vi "Open.vi"(9 "force":dbl, 10 "Lever":refnum<class "Lever.lvclass">, 11 "Box in":refnum<class "Box.lvclass">) -> (3 "Box out":refnum<class "Box.lvclass">)   [LabVIEW 2023, in "Box.lvclass"]
uses:
  Box.lvclass
  c:/dev/_r/4/eng/lv-core/lvpostprocessingd/lv_mc_x86_64/dist_i386/examples/Object-Oriented Programming/Basic Interfaces/Pryable/Pryable.lvclass
  Lever/Lever.lvclass
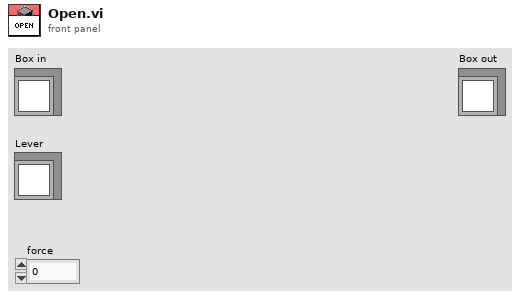
[diagram p1: front panel]
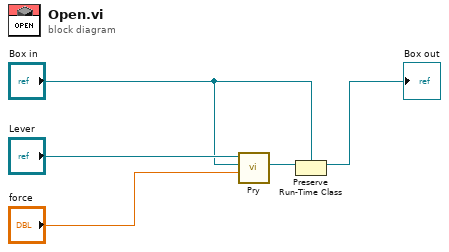
[diagram p0: block diagram]
diagram:
  n1 = call "Pry.vi"("force"="force", "Pryable in"="Box in", "Lever in"="Lever") -> ("Pryable out"=w4:refnum<class "Box.lvclass">)  [unwired: 8 in]
  n2 = Preserve Run-Time Class(object in=w4, 2:"Box in") -> (object out=→"Box out":refnum<class "Box.lvclass">)  [unwired: 1 in, 1 out]
